vi "obtain_timestamp.vi"(4 "Bit offset (1200)":i32=1200, 5 "LiDAR raw data":string) -> (2 "Timestamp (us)":u32)   [LabVIEW 2019, in "Lib_Simx.lvlib"]
doc: "Obtains timestamp (byte 1200) in microseconds from the raw LiDAR stream (1206 bytes)."
uses:
  Lib_Simx.lvlib
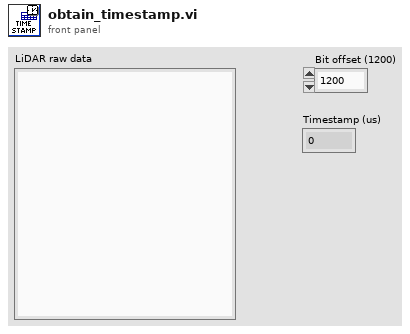
[diagram p1: front panel]
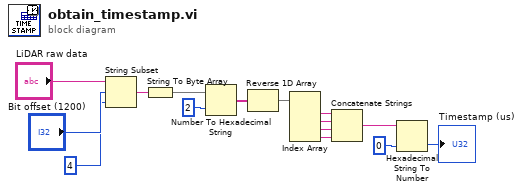
[diagram p0: block diagram]
diagram:
  n1 = String Subset(string="LiDAR raw data", offset (0)="Bit offset (1200)", length (rest)=4 ("length (rest)")) -> (substring=w4:string)
  n2 = String To Byte Array(string=w4) -> (unsigned byte array=w7:u8[])
  n3 = Number To Hexadecimal String(1:i16 2 ("width (-)"), 2:w7) -> (0:w8:string[])
  n4 = Reverse 1D Array(array=w8) -> (reversed array=w9:string[])
  n5 = Index Array(array=w9) -> (element #1=w10:string, element #2=w11:string, element #3=w13:string, element #4=w14:string)  [unwired: 4 in]
  n6 = Concatenate Strings(w10, w11, w13, w14) -> (w2:string)
  n7 = Hexadecimal String To Number(string=w2, default (0uL)=u32 0 ("default (0 U32)")) -> (number=→"Timestamp (us)":u32)  [unwired: 1 in, 1 out]
